vi "1K_filter.vi"(0 "Frecuencia de corte alto":dbl=1050.0 format="%0.2f", 1 "Frecuencia de  corte bajo":dbl=950.0 format="%0.2f", 2 "filter type":T1=enum."Bandstop", 3 "Ventana":T2 items=["Rectangle"=0, "Hanning"=1, "Hamming"=2, "Blackman-Harris"=3, "Exact Blackman"=4, "Blackman"=5, "Flat Top"=6, "4 Term B-Harris "=7, "7 Term B-Harris"=8, "Low Sidelobe"=9, "Blackman Nuttall"=11, "Triangle"=30, "Bartlett-Hanning"=31, "Bohman"=32, "Parzen"=33, "Welch"=34, "Kaiser"=60, "Dolph-Chebyshev"=61, "Gaussian"=62], 4 "Cantidad de Taps":i32=3001 min=1) -> (5 "FIR Windowed Coefficients":dbl[](array[numeric]))   [LabVIEW 2018]
uses:
  <vilib>/Analysis/4window.llb/windowTd.ctl
  <vilib>/Analysis/3filter.llb/Filter Passband Type.ctl
  <vilib>/Analysis/NI_AALBase.lvlib
  <vilib>/Analysis/NI_AALPro.lvlib
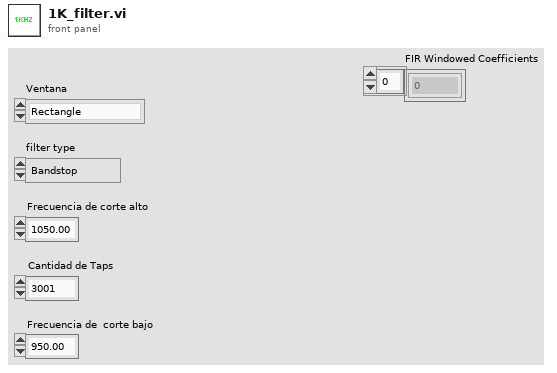
[diagram p1: front panel]
types:
  T1 = typedef "NI_AALBase.lvlib/Filter Passband Type.ctl" = enum32{"Lowpass", "Highpass", "Bandpass", "Bandstop"}
  T2 = typedef "NI_AALPro.lvlib/windowTd.ctl" = u32
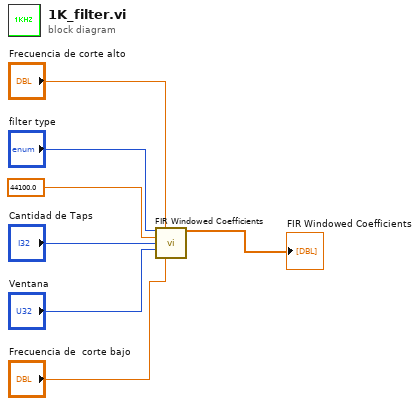
[diagram p0: block diagram]
diagram:
  n1 = call <vilib>:"FIR Windowed Coefficients.vi"("filter type"="filter type", "high cutoff freq: fh"="Frecuencia de corte alto", "sampling freq: fs"=44100.0, "taps"="Cantidad de Taps", "window"="Ventana", "low cutoff freq: fl"="Frecuencia de  corte bajo") -> ("FIR Windowed Coefficients"=→"FIR Windowed Coefficients":dbl[])  [unwired: 8 in, 1 out]
